vi "Unary RouteGuide Test.vi"() -> ()   [LabVIEW 2019, in "route_guide_client.lvlib"]
uses:
  route_guide_client.lvlib
  RPC Messages/routeguide_Point.ctl
  RPC Messages/routeguide_Feature.ctl
  <vilib>/gRPC/LabVIEW gRPC Library/grpc-lvsupport-release.lvlib
panel:
  out "error out":errorcluster
  in  "Server Address":string="localhost:50051"
  out "Response Data":T1
  in  "Request Data":T2={"latitude"=4, "longitude"=5}
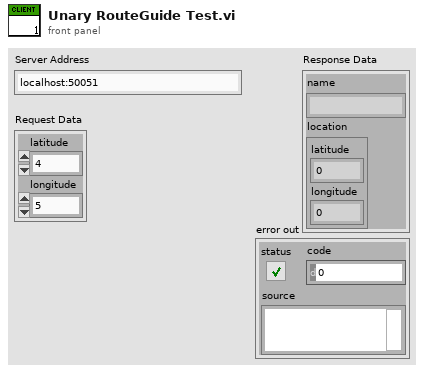
[diagram p1: front panel]
types:
  T1 = typedef "route_guide_client.lvlib/routeguide_Feature.ctl" = cluster{"name":string, "location":T2}
  T2 = typedef "route_guide_client.lvlib/routeguide_Point.ctl" = cluster{"latitude":i32, "longitude":i32}
  T3 = typedef "grpc-lvsupport-release.lvlib/grpcId.ctl" = u64
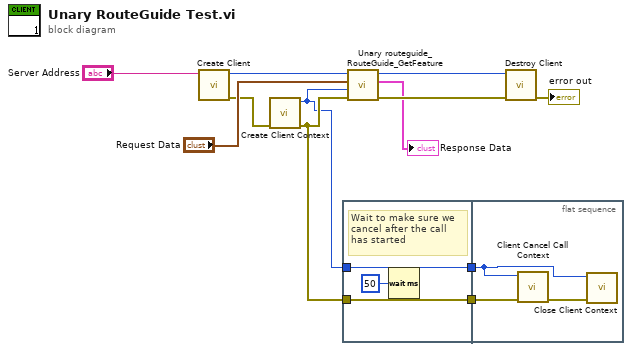
[diagram p0: block diagram]
diagram:
  n1 = call "Create Client.vi"("address"="Server Address") -> ("error out"=w5:errorcluster, "gRPC ID Out"=w12:T3)  [unwired: 9 in]
  n2 = call <vilib>:"Create Client Context.vi"("error in (no error)"=w5) -> ("error out"=w4:errorcluster, "ContextID out"=w3:T3)  [unwired: 9 in]
  n3 = flat-sequence {
    tunnel: w3 -> [w14]
    tunnel: w4 -> [w15]
    tunnel: [w15] -> w2
    tunnel: [w14] -> w1
    tunnel: w2 -> [w18]
    tunnel: w1 -> [w16]
    frame #0 {
      # "Wait to make sure we cancel after the call has started"
      n4 = Wait (ms)(milliseconds to wait=u32 50) -> ()  [unwired: 1 out]
    }
    frame #1 {
      n5 = call <vilib>:"Client Cancel Call Context.vi"("error in"=w18, "Call ID in"=w16) -> ("error out"=w17:errorcluster)  [unwired: 9 in]
      n6 = call <vilib>:"Close Client Context.vi"("error in (no error)"=w17, "ContextID"=w16) -> ()  [unwired: 9 in, 1 out]
    }
  }
  n7 = call "Unary routeguide_RouteGuide_GetFeature.vi"("error in"=w4, "contextId"=w3, "Request Data"="Request Data", "gRPC ID"=w12) -> ("error out"=w11:errorcluster, "Response Data"=→"Response Data":T1, "gRPC ID out"=w10:T3)  [unwired: 5 in]
  n8 = call "Destroy Client.vi"("error in"=w11, "gRPC ID"=w10) -> ("error out"=→"error out":errorcluster)  [unwired: 9 in]
